vi "RefreshDevice.vi"(8 "error in (no error)":errorcluster, 11 "Serial Controller in":refnum<class "Serial Controller.lvclass">) -> (0 "error out":errorcluster, 3 "Serial Controller out":refnum<class "Serial Controller.lvclass">)   [LabVIEW 2011, in "Serial Controller.lvclass"]
uses:
  Serial Controller.lvclass
  Serial Controller.lvclass/Serial Controller.ctl
panel:
  in  "RefreshTimes":i32=10
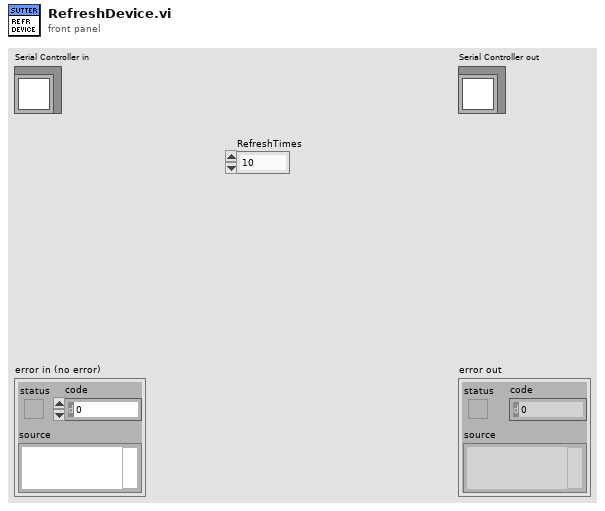
[diagram p1: front panel]
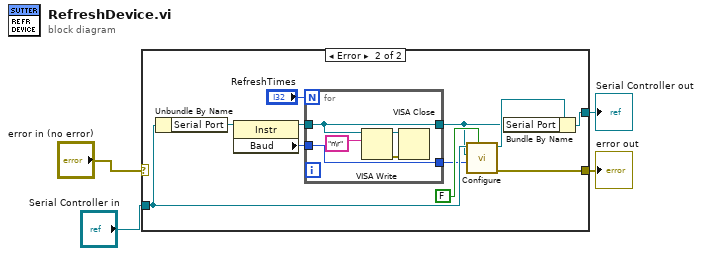
[diagram p0: block diagram]
diagram:
  n1 = case shown="Error" "error in (no error)" {
    selector: "error in (no error)" -> [w6 _]
    tunnel: [w6 w8] -> w3
    tunnel: [w5 w15] -> w1
    tunnel: "Serial Controller in" -> [w5 w13]
    frame No Error {
    }
    frame Error {
      n2 = Unbundle By Name(w13) -> ("Serial Port"=w14:refnum<visa-resource-name>)
      n3 = property class="Instr"(reference=w14) -> (reference out=w16:refnum<visa-resource-name>, "Baud"=w17:u32)  [unwired: 1 in, 1 out]
      n4 = for {
        N: "RefreshTimes" -> [_]
        tunnel: w16 -> [w18]
        tunnel: w17 -> [w21]
        tunnel: [w21] -> w10
        tunnel: [w18] -> w9
        n5 = VISA Write(VISA resource name=w18, write buffer="n\r") -> (VISA resource name out=w22:refnum<visa-resource-name>, error out=w20:errorcluster)  [unwired: 1 in, 1 out]
        n6 = VISA Close(VISA resource name=w22, error in (no error)=w20) -> ()  [unwired: 1 out]
      }
      n7 = call-dynamic "Configure.vi"("Reset"=FALSE, "baud rate (9600)"=w10, "VISA resource name"=w9, "Serial Controller in"=w13) -> ("error out"=w8:errorcluster, "Serial Controller out"=w12:refnum<class "Serial Controller.lvclass">)  [unwired: 6 in]
      n8 = Bundle By Name(cluster=w12, "Serial Port"=w9) -> (w15:refnum<class "Serial Controller.lvclass">)
    }
  }
  "error out" <- w3
  "Serial Controller out" <- w1
